vi "Update Z Scale Marker Values.vi"(8 "error in":errorcluster, 10 "Z Scale.Marker Values[]":cluster{dbl, u32}[](array[cluster]), 11 "Base Graph in":refnum<class "Base Graph.lvclass">) -> (0 "error out":errorcluster, 3 "Base Graph out":refnum<class "Base Graph.lvclass">)   [LabVIEW 2025, in "Base Graph.lvclass"]
uses:
  Base Graph.lvclass
  Base Graph.lvclass/Base Graph.ctl
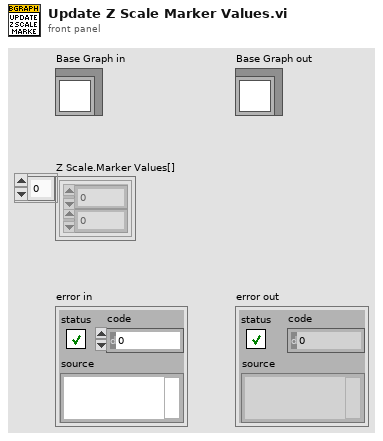
[diagram p1: front panel]
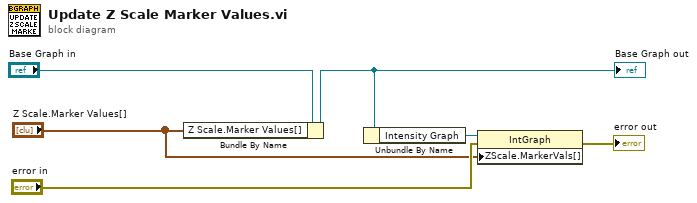
[diagram p0: block diagram]
diagram:
  n1 = Bundle By Name(cluster="Base Graph in", "Z Scale.Marker Values[]"="Z Scale.Marker Values[]") -> (w2:refnum<class "Base Graph.lvclass">)
  "Base Graph out" <- w2
  n2 = Unbundle By Name(w2) -> ("Intensity Graph"=w4:refnum<vi>)
  n3 = property class="IntGraph"(reference=w4, error in="error in", "ZScale.MarkerVals[]"="Z Scale.Marker Values[]") -> (error out=→"error out":errorcluster)  [unwired: 1 out]
